vi "Main.vi"() -> ()   [LabVIEW 2013]
panel:
  out "Voltage":dbl
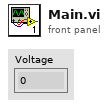
[diagram p1: front panel]
types:
  T1 = typedef "KNR3 Reference.ctl" = cluster{"FPGA Session":refnum<class "FPGA Interface Base.lvclass">, "Resource":T2}
  T2 = typedef "Resource.ctl" = enum16{"KNRm_DDRC", "KNRm_DDDD", "KNRm_DDDR", "KNRm_DDDC", "KNR"}
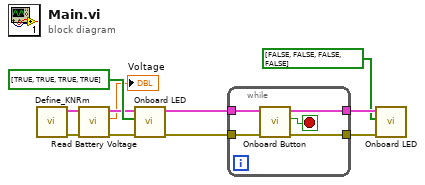
[diagram p0: block diagram]
diagram:
  n1 = call "Define_KNRm.vi"() -> ("error out"=w4:errorcluster, "KNR out"=w5:T1)  [unwired: 10 in]
  n2 = call <userlib>:"Read Battery Voltage.vi"("error in (no error)"=w4, "KNR in"=w5) -> ("error out"=w7:errorcluster, "Voltage"=→"Voltage":dbl, "KNR out"=w6:T1)  [unwired: 7 in]
  n3 = call <userlib>:"Onboard LED.vi"("error in (no error)"=w7, "LED List"=bool[] [TRUE, TRUE, TRUE, TRUE], "KNR in"=w6) -> ("error out"=w1:errorcluster, "KNR out"=w2:T1)  [unwired: 7 in]
  n4 = while {
    tunnel: w2 -> [w16]
    tunnel: w1 -> [w15]
    tunnel: [w13] -> w10
    tunnel: [w12] -> w9
    stop <- w14 stop-if-true
    n5 = call <userlib>:"Onboard Button.vi"("error in (no error)"=w15, "KNR in"=w16) -> ("error out"=w12:errorcluster, "value"=w14:bool, "KNR out"=w13:T1)  [unwired: 7 in]
  }
  n6 = call <userlib>:"Onboard LED.vi"("error in (no error)"=w9, "LED List"=bool[] [FALSE, FALSE, FALSE, FALSE], "KNR in"=w10) -> ()  [unwired: 7 in, 2 out]
